vi "Add Always Excluded.vi"(8 "error in (no error)":errorcluster, 10 "ProjectItem Refnum":refnum<vi>, 11 "SDIST in":refnum<class "NI_AB_API_SDIST.lvclass">) -> (0 "error out":errorcluster, 3 "SDIST out":refnum<class "NI_AB_API_SDIST.lvclass">)   [LabVIEW 2020, in "NI_AB_API_SDIST.lvclass"]
uses:
  <vilib>/AppBuilder/AB_API/SDIST/NI_AB_API_SDIST.lvclass
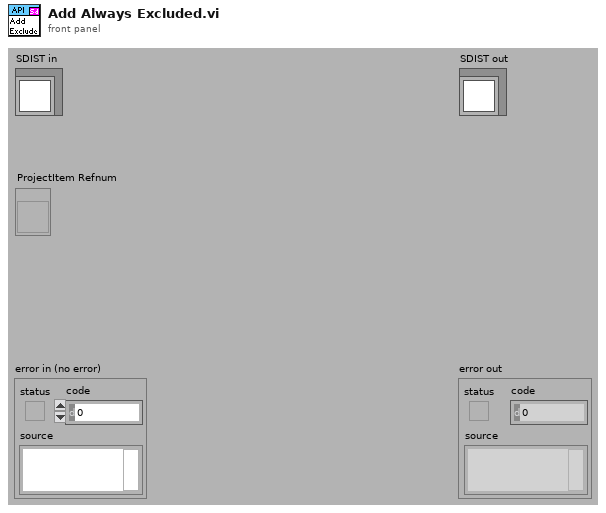
[diagram p1: front panel]
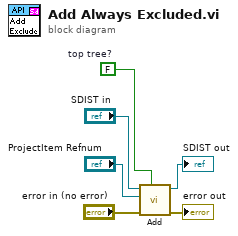
[diagram p0: block diagram]
diagram:
  w2 = FALSE  # top tree?
  n1 = call-dynamic "Add.vi"("top tree? (true)"=w2, "error in (no error)"="error in (no error)", "ProjectItem Refnum"="ProjectItem Refnum", "SDIST in"="SDIST in") -> ("error out"=→"error out":errorcluster, "SDIST out"=→"SDIST out":refnum<class "NI_AB_API_SDIST.lvclass">)  [unwired: 6 in]
